vi "5.1.vi"() -> ()   [LabVIEW 2017]
panel:
  out "数组（最后n个元素置于前端）":dbl[](array[numeric])
  out "数组":dbl[](array[numeric])
  out "反转的数组":dbl[](array[numeric])
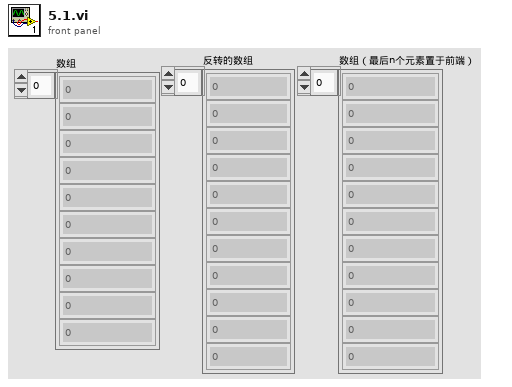
[diagram p1: front panel]
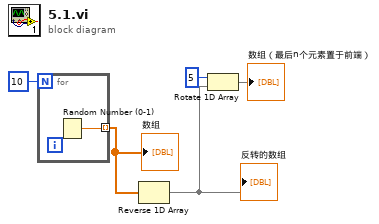
[diagram p0: block diagram]
diagram:
  n1 = for {
    N: 10 -> [_]
    tunnel: [w6] -> w4 mode=indexing
    n2 = Random Number (0-1)() -> (number: 0 to 1=w6:dbl)
  }
  "数组" <- w4
  n3 = Reverse 1D Array(array=w4) -> (reversed array=w2:dbl[])
  "反转的数组" <- w2
  n4 = Rotate 1D Array(1:w2, 2:5 ("n")) -> (0:→"数组（最后n个元素置于前端）":dbl[])
